vi "DestroyModuleBroadcasts.vi"(8 "error in (no error)":errorcluster, 11 "NewTemplate in":refnum<class "TitleBar.lvclass">) -> (0 "error out":errorcluster, 3 "NewTemplate out":refnum<class "TitleBar.lvclass">)   [LabVIEW 2024, in "TitleBar.lvclass"]
uses:
  TitleBar.lvclass
  TitleBar.lvclass/TitleBar.ctl
  RQMHCore/ModuleCore/Module.lvclass
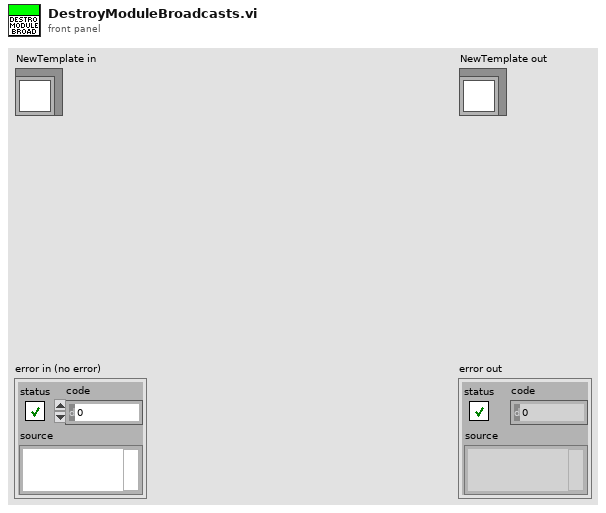
[diagram p1: front panel]
types:
  T1 = typedef "TitleBar.lvclass/Broadcast Events--cluster.ctl" = cluster{"Stopped":refnum<user-event>, "Maximise":refnum<user-event>, "Minimise":refnum<user-event>, "ClosePress":refnum<user-event>}
  T2 = typedef "TitleBar.lvclass/Request Events--cluster.ctl" = cluster{"Do Something":refnum<user-event>, "AddTopLevelVI":refnum<user-event>}
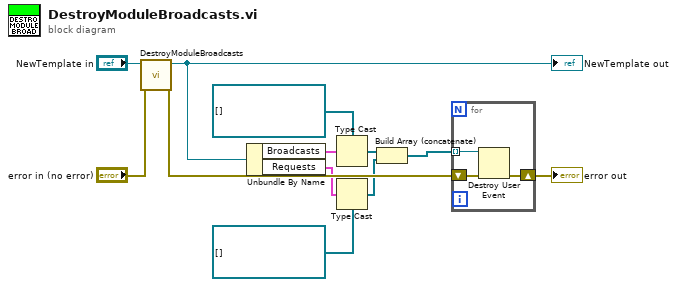
[diagram p0: block diagram]
diagram:
  n1 = call-parent "DestroyModuleBroadcasts.vi"("error in (no error)"="error in (no error)", "JQMHModule in"="NewTemplate in") -> ("error out"=w6:errorcluster, "JQMHModule out"=w8:refnum<class "TitleBar.lvclass">)  [unwired: 8 in]
  "NewTemplate out" <- w8
  n2 = Unbundle By Name(w8) -> ("Broadcasts"=w11:T1, "Requests"=w4:T2)
  n3 = Type Cast(type=refnum<user-event>[] [] ("NewControl5"), x=w11) -> (*(type *) &x=w2:refnum<user-event>[])
  n4 = Type Cast(type=refnum<user-event>[] [] ("NewControl5"), x=w4) -> (*(type *) &x=w3:refnum<user-event>[])
  n5 = Build Array (concatenate)(w2, w3) -> (w1:refnum<user-event>[])
  n6 = for {
    tunnel: w1 -> [w15] mode=indexing
    shift-right: [w13] -> w10
    shift-left: w6 -> [w14]
    n7 = Destroy User Event(user event=w15, error in=w14) -> (error out=w13:errorcluster)
  }
  "error out" <- w10
